vi "Pre Launch Init.vi"(11 "server in":refnum<class "server.lvclass">) -> (0 "error out":errorcluster, 3 "server out":refnum<class "server.lvclass">)   [LabVIEW 2016, in "server.lvlib" / "server.lvclass"]
doc: "(<B>Filename</B>: Actor Framework.lvlib:Actor.lvclass:Pre Launch Init.vi)\n\nDefines behavior that occurs after the Launch Nested Actor method is invoked but before the actor's Actor Core method begins running.\n\nBy default, this method does nothing. A descendant class may override it to define behavior."
uses:
  server.lvclass
  server.lvclass/server.ctl
  <vilib>/ActorFramework/Actor/Actor.lvclass
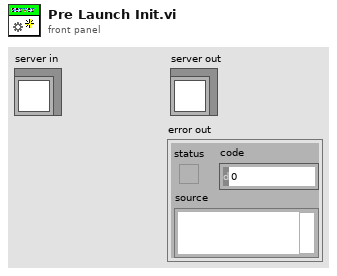
[diagram p1: front panel]
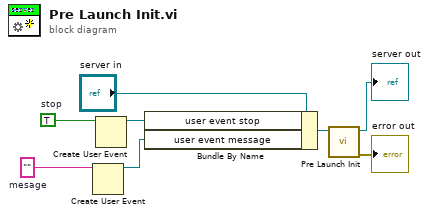
[diagram p0: block diagram]
diagram:
  w2 = ""  # mesage
  w5 = TRUE  # stop
  n1 = Create User Event(user event datatype=w2) -> (user event=w1:refnum<user-event>)  [unwired: 1 in, 1 out]
  n2 = Create User Event(user event datatype=w5) -> (user event=w4:refnum<user-event>)  [unwired: 1 in, 1 out]
  n3 = Bundle By Name(cluster="server in", "user event stop"=w4, "user event message"=w1) -> (w3:refnum<class "server.lvclass">)
  n4 = call-parent "Pre Launch Init.vi"("Actor in"=w3) -> ("error out"=→"error out":errorcluster, "Actor out"=→"server out":refnum<class "server.lvclass">)  [unwired: 9 in]
